vi "二维数组的chart 与 graph的区别 和图像叠加.vi"() -> ()   [LabVIEW 2023]
panel:
  out "Waveform Chart 3":dbl[][](graph)
  out "chart array":dbl[][](array[numeric])
  out "graph array":dbl[][](array[numeric])
  out "Waveform Graph 2":dbl[][](graph)
  out "Waveform Chart 2":dbl[][](graph)
  out "Waveform Graph":dbl[](graph)
  out "Waveform Chart":dbl[](graph)
  # "二维数组的chart 与 graph的区别 和图像叠加"
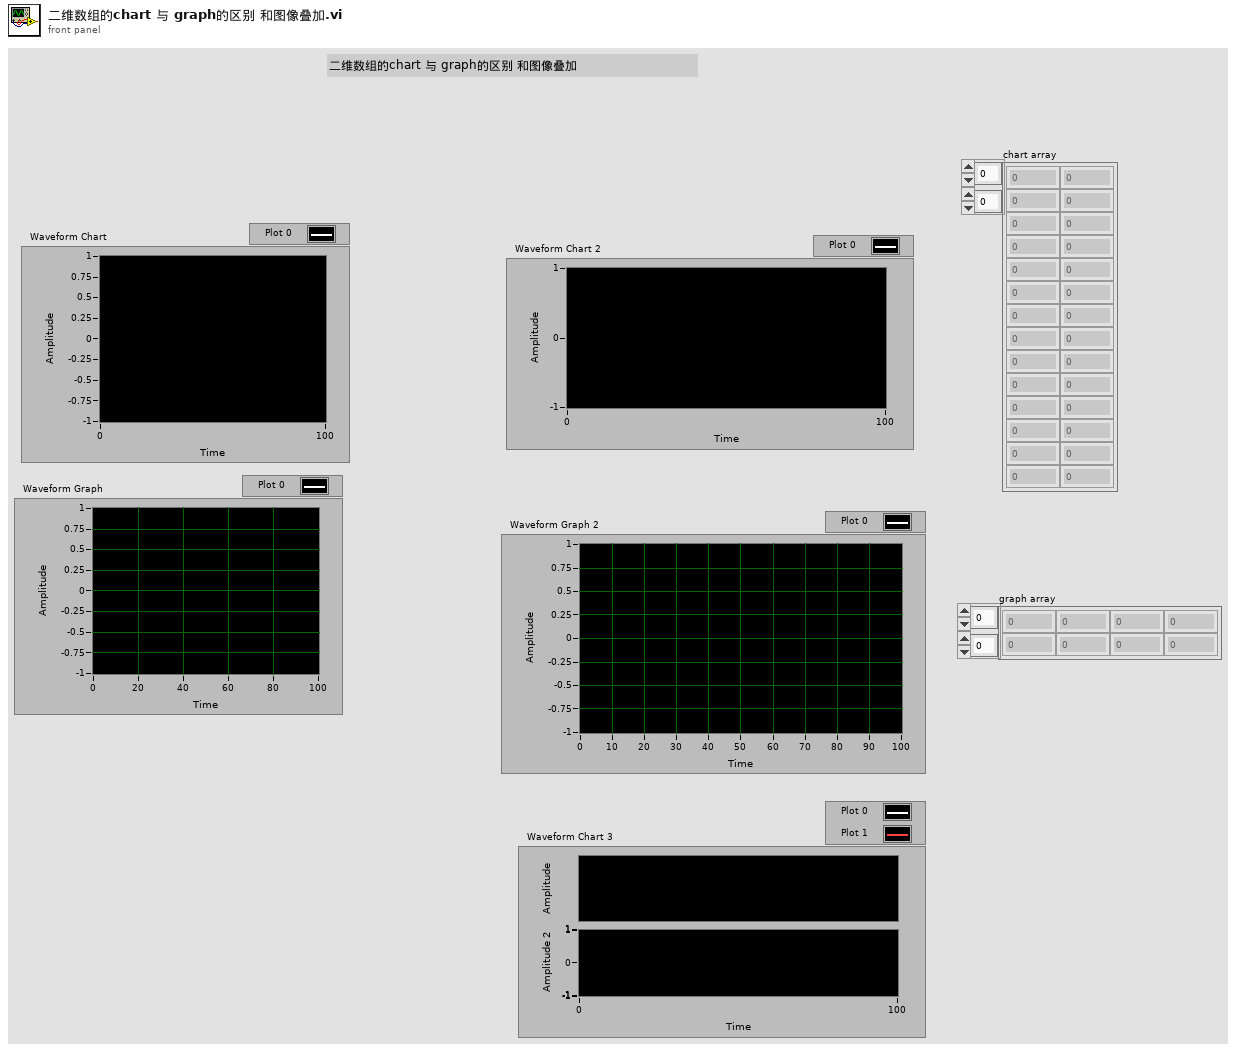
[diagram p1: front panel]
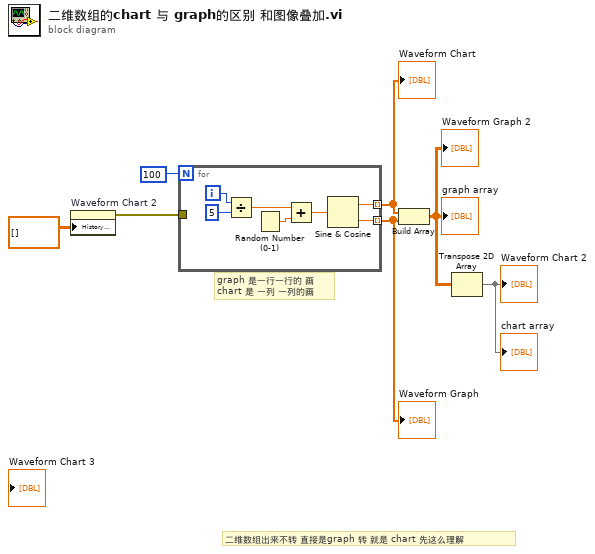
[diagram p0: block diagram]
diagram:
  # "二维数组出来不转 直接是graph 转 就是 chart 先这么理解"
  # "graph 是一行一行的 画\nchart 是 一列 一列的画"
  n1 = property on="Waveform Chart 2" class="WFChart (strict)"("History Data"=dbl[][] []) -> (error out=w4:errorcluster)  [unwired: 2 in, 1 out]
  n2 = for {
    N: 100 -> [_]
    tunnel: [w9] -> w6 mode=indexing
    tunnel: [w8] -> w5 mode=indexing
    tunnel: w4 -> [_]
    i -> [w14]
    n3 = Divide(x=w14, y=5) -> (x/y=w12:dbl)
    n4 = Random Number (0-1)() -> (number: 0 to 1=w11:dbl)
    n5 = Add(x=w12, y=w11) -> (x+y=w10:dbl)
    n6 = Sine & Cosine(0:w10) -> (1:w9:dbl, 2:w8:dbl)
  }
  "Waveform Chart" <- w6
  "Waveform Graph" <- w5
  n7 = Build Array(w6, w5) -> (w2:dbl[][])
  "Waveform Graph 2" <- w2
  "graph array" <- w2
  n8 = Transpose 2D Array(2D array=w2) -> (transposed array=→"Waveform Chart 2" →"chart array":dbl[][])
